vi "configuration UI.vi"() -> ()   [LabVIEW 2013, in "tag bus processing plugin editor node.lvclass"]
uses:
  tag bus processing plugin editor node.lvclass
  <vilib>/CEF_TreeControl/Node/NodeRef.ctl
  <vilib>/CEF_TreeControl/Node/NISE_CEF_Node.lvclass
  <vilib>/NI/AMC/Message Queue.ctl
  <vilib>/NI/AMC/Message.ctl
  <vilib>/NI/Tools/Keyed Array/KeyedArray.ctl
  <vilib>/CEF_TreeControl/Node/UserEventRef.ctl
  <vilib>/CEF_TreeControl/Controls/EventCluster.ctl
  module/configuration/tag bus processing plugin module configuration.lvclass
  module/configuration/processing channels.ctl
  <vilib>/NI/Tag Bus Module Framework/channel/TBM channel.lvclass
  <vilib>/NI/Tag Bus Module Framework/root configuration/TBM configuration.lvclass/TBM configuration.ctl
  Configuration Editor/Classes/Engine Parent/Engine Parent Editor Node.lvclass
  <vilib>/NI/Tag Bus Module Framework/root configuration/Read instance name.vi
  Configuration Editor/Classes/Module editor node/Read Module Configuration.vi
  <vilib>/NI/Tag Bus Module Framework/root configuration/create GUID.vi
  <vilib>/NI/Tag Bus Module Framework/module configuration/TBM module configuration.lvclass
  <vilib>/NI/Module Execution Interface/Engine Configuration/engine configuration.lvclass
  <vilib>/CEF_TreeControl/NISE_CEF_TreeControl.lvlib
  <vilib>/NI/Tools/Keyed Array/Tools_KeyedArray.lvlib
  <vilib>/NI/AMC/AMC.lvlib
panel:
  in  "Tab Control":enum32{"Control Configuration"}(tab)
  in  "delete":bool
  in  "add":bool
  in  "Result Tag":u16(ring)
  in  "Parameter Tag":u16(ring)
  in  "Functions":i32(listbox)
  in  "user event":T1
  in  "main queue":T2
  in  "node ref":T3
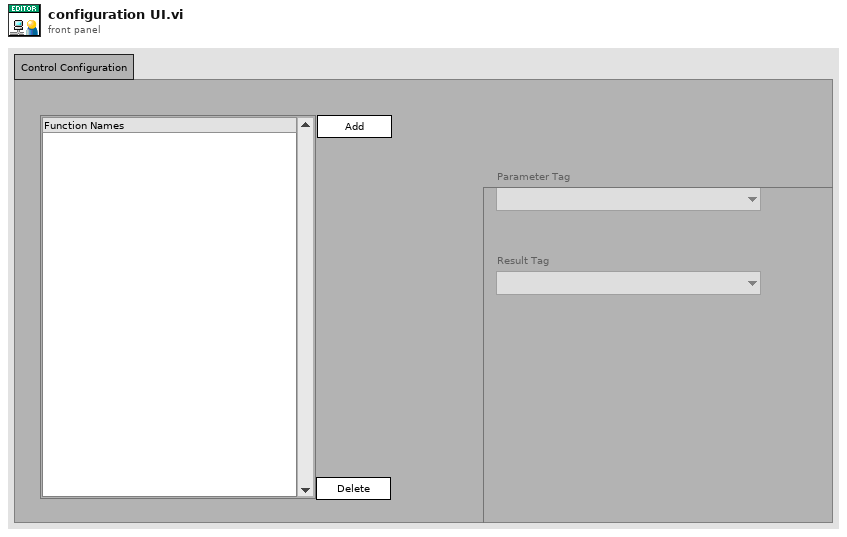
[diagram p1: front panel]
types:
  T1 = typedef "NISE_CEF_Node.lvclass/UserEventRef.ctl" = refnum<user-event>
  T2 = typedef "AMC.lvlib/Message Queue.ctl" = refnum<queue>
  T3 = typedef "NISE_CEF_Node.lvclass/NodeRef.ctl" = refnum<data-value>
  T4 = typedef "tag bus processing plugin module configuration.lvclass/processing channels.ctl" = cluster{"parameter":refnum<class "TBM channel.lvclass">, "result":refnum<class "TBM channel.lvclass">}
  T5 = typedef "NISE_CEF_TreeControl.lvlib/EventCluster.ctl" = cluster{"command":string, "data":string}
  T6 = enum8{"Enabled", "Disabled", "Disabled and Grayed Out"}
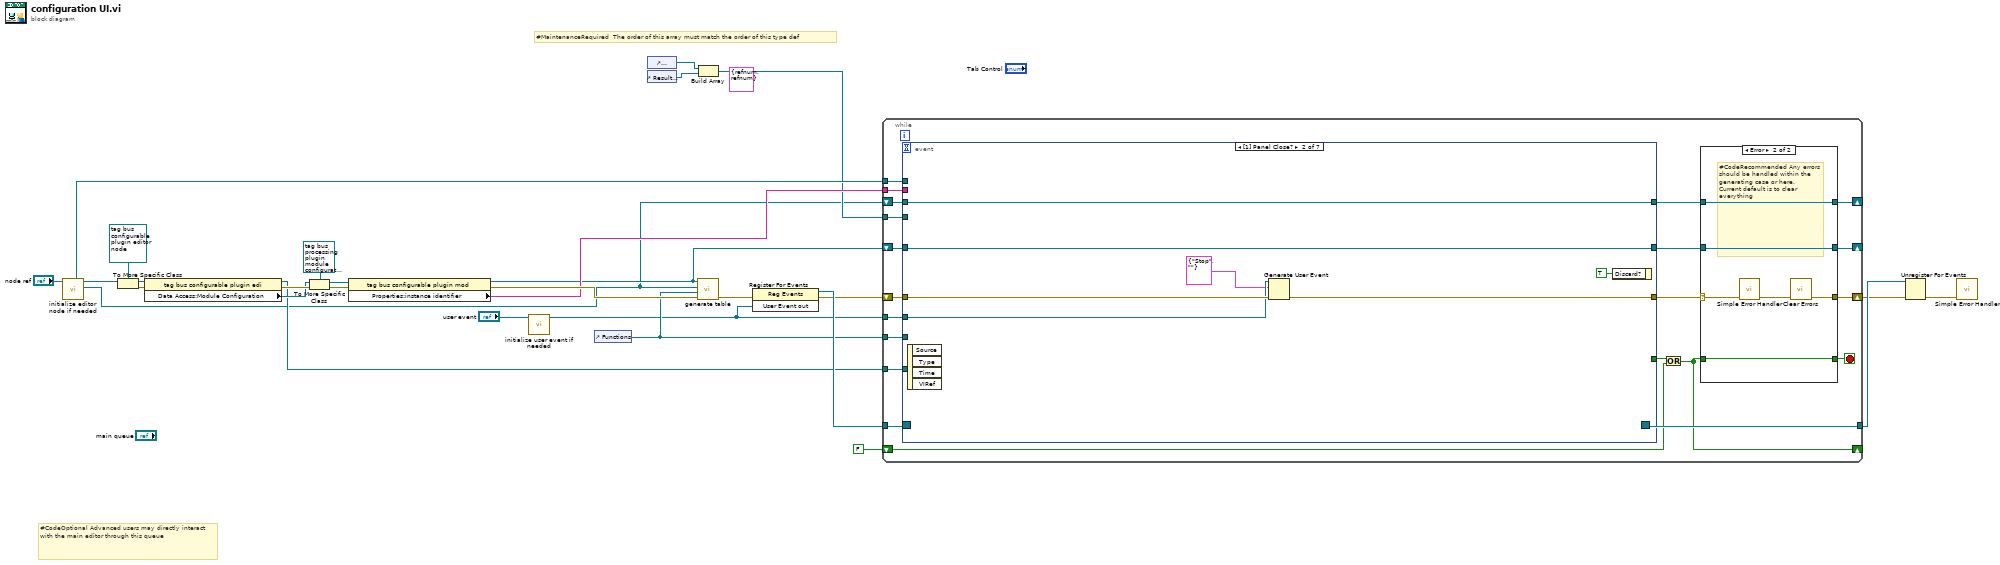
[diagram p0: block diagram]
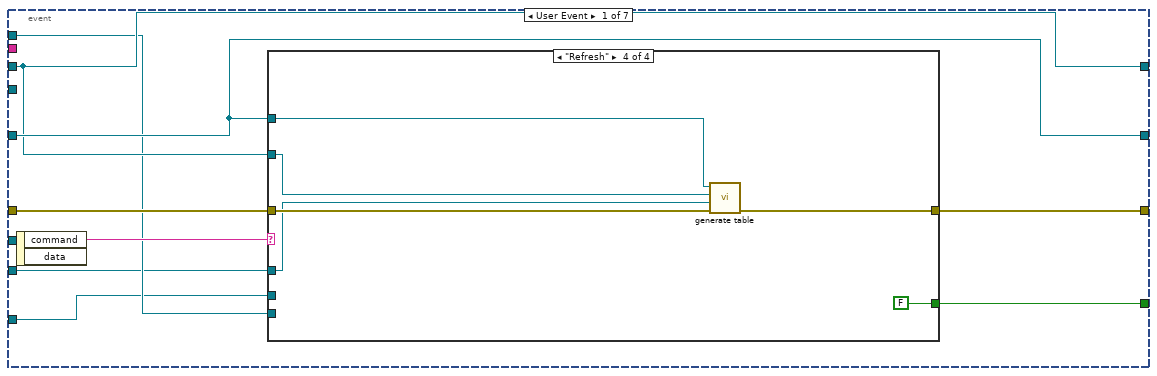
[diagram p3: hidden frame]
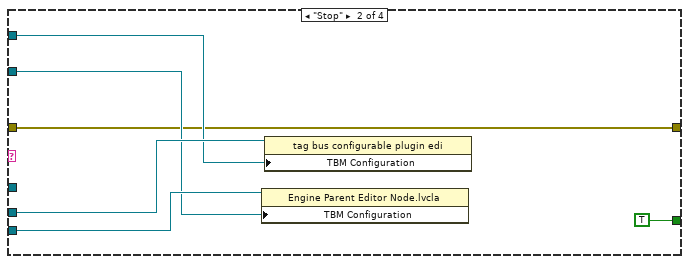
[diagram p5: hidden frame]
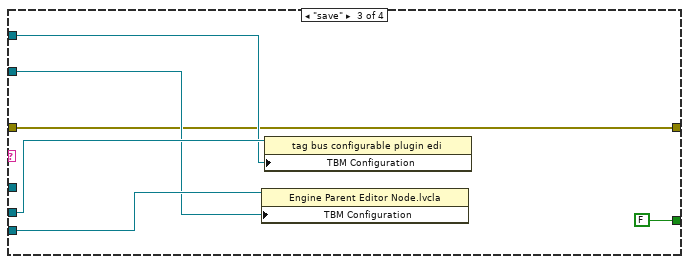
[diagram p6: hidden frame]
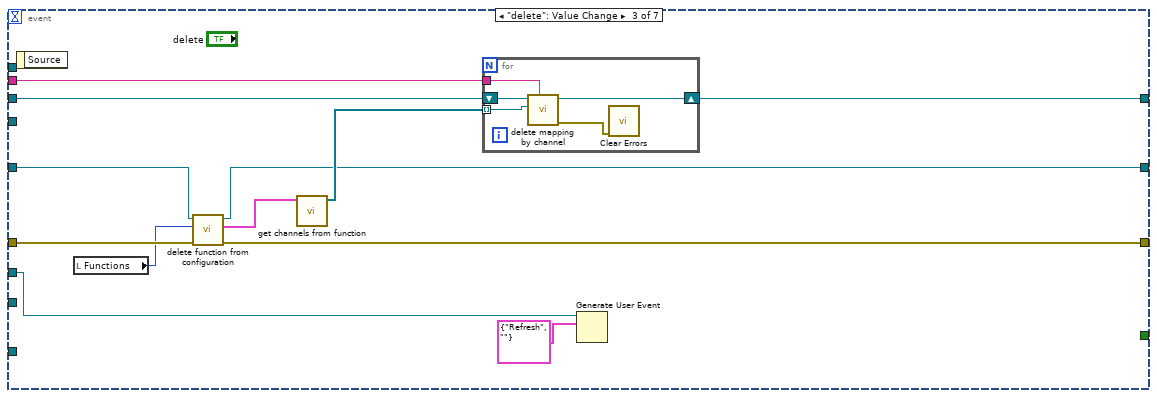
[diagram p7: hidden frame]
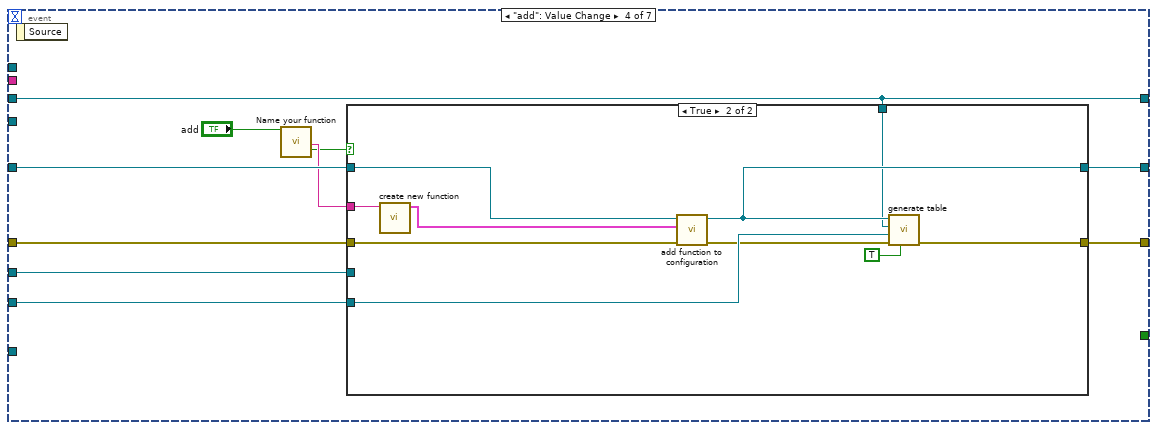
[diagram p8: hidden frame]
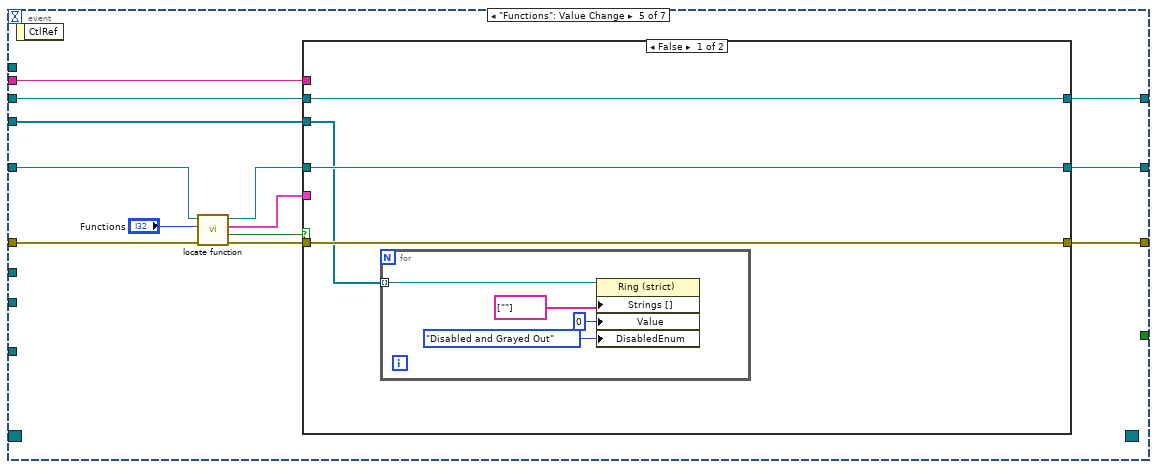
[diagram p10: hidden frame]
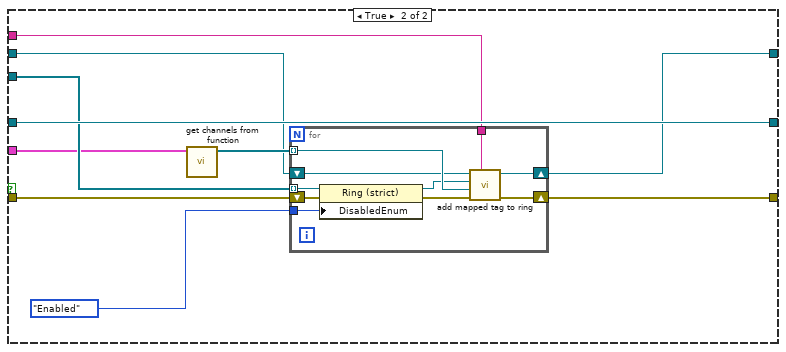
[diagram p11: hidden frame]
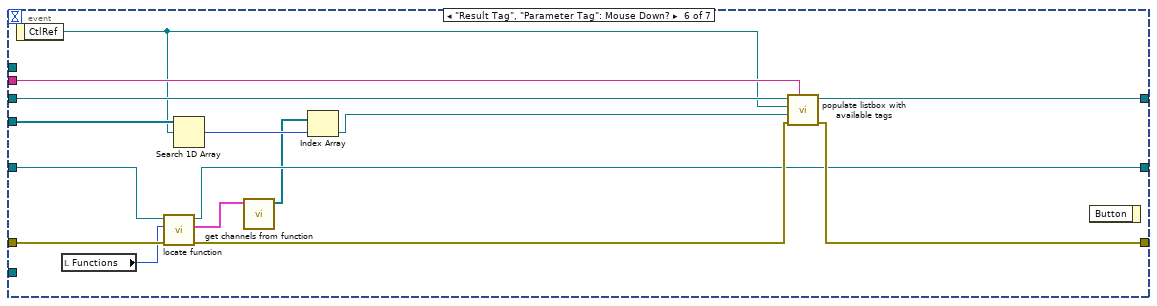
[diagram p12: hidden frame]
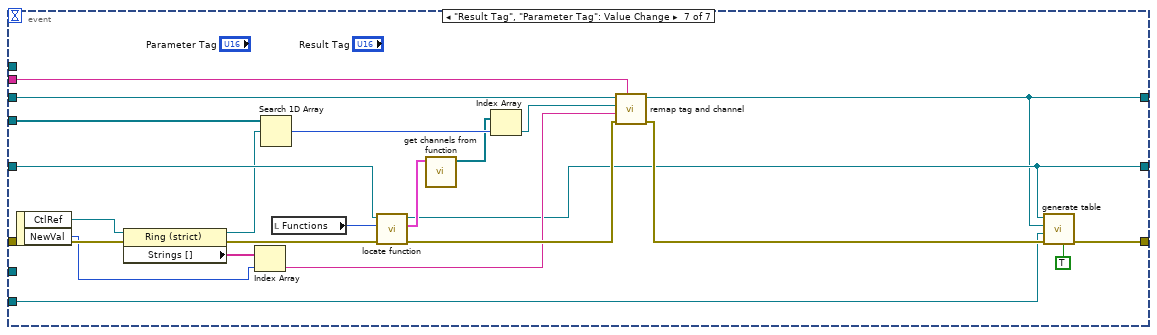
[diagram p13: hidden frame]
diagram:
  (unwired) T4 {"parameter"=refnum, "result"=refnum} ("processing function")
  # "#MaintenanceRequired  The order of this array must match the order of this type def"
  # "#CodeOptional Advanced users may directly interact with the main editor through this queue"
  n1 = call "initialize editor node if needed.vi"("editor node in"="node ref") -> ("Engine Configuration"=w1:refnum<class "engine configuration.lvclass">, "editor node out"=w21:T3, "engine"=w19:refnum<data-value>)  [unwired: 8 in]
  n2 = To More Specific Class(target class=refnum<data-value> refnum ("data value reference"), reference=w21) -> (specific class reference=w17:refnum<data-value>, error out=w16:errorcluster)  [unwired: 1 in]
  n3 = property class="tag bus configurable plugin edi"(reference=w17, error in=w16) -> (reference out=w7:refnum<data-value>, error out=w15:errorcluster, "Data Access:Module Configuration"=w14:refnum<class "TBM module configuration.lvclass">)
  n4 = To More Specific Class(target class=refnum<class "tag bus processing plugin module configuration.lvclass"> refnum ("tag bus configurable plugin module configuration"), reference=w14, error in=w15) -> (specific class reference=w11:refnum<class "tag bus processing plugin module configuration.lvclass">, error out=w12:errorcluster)
  n5 = property class="tag bus configurable plugin mod"(reference=w11, error in=w12) -> (reference out=w2:refnum<class "tag bus processing plugin module configuration.lvclass">, error out=w10:errorcluster, "Properties:instance identifier"=w9:string)
  n6 = call "initialize user event if needed.vi"("User Event in"="user event") -> ("User Event out"=w3:T1)  [unwired: 10 in]
  n7 = control-ref of="Functions"() -> (w8:refnum<vi>)
  n8 = control-ref of="Parameter Tag"() -> (w6:refnum<vi>)
  n9 = control-ref of="Result Tag"() -> (w5:refnum<vi>)
  n10 = call "generate table.vi"("error in"=w10, "listbox"=w8, "engine configuration in"=w1, "tag bus configurable plugin module configuration in"=w2) -> ("error out"=w24:errorcluster)  [unwired: 7 in]
  n11 = Build Array(w6, w5) -> (w4:refnum<vi>[])
  n12 = register-events(error in=w24, w3) -> (reference out=w29:refnum<event-registration>, error out=w23:errorcluster)  [unwired: 1 in]
  n13 = while {
    tunnel: w29 -> [w50]
    tunnel: [w49] -> w28
    shift-right: [w42] -> w27
    shift-left: w23 -> [w48]
    shift-right: [w44] -> _
    shift-left: FALSE -> [w43]
    shift-right: [w38] -> _
    shift-left: w1 -> [w41]
    shift-right: [w37] -> _
    shift-left: w2 -> [w40]
    tunnel: w9 -> [w35]
    tunnel: w8 -> [w34]
    tunnel: w4 -> [w33]
    tunnel: w7 -> [w32]
    tunnel: w19 -> [w31]
    tunnel: w3 -> [w30]
    stop <- w46 stop-if-true
    n14 = event shown="[1] Panel Close?" {
      selector: w50 -> [_ _ _ _ _ _ _]
      dyn-events: [_ _ _ _ _ _ _] -> w49
      timeout: _ -> [_ _ _ _ _ _ _]
      tunnel: [w66 _ _ _ _ _ _] -> w45
      tunnel: [w69 w92 w100 w122 w141 w187 w202] -> w47
      tunnel: w48 -> [w68 w95 w107 w119 w147 w186 w213]
      tunnel: [w64 w94 w98 w113 w138 w189 w191] -> w39
      tunnel: w41 -> [w64 w94 w103 w113 w137 w190 w210]
      tunnel: [w65 w93 w99 w121 w140 w183 w192] -> w36
      tunnel: w40 -> [w65 w93 w105 w118 w146 w184 w205]
      tunnel: w35 -> [_ _ w101 _ w136 w188 w209]
      tunnel: w34 -> [w61 _ _ w120 _ _ w201]
      tunnel: w33 -> [_ _ _ _ w135 w181 w198]
      tunnel: w32 -> [w62 _ _ _ _ _ _]
      tunnel: w31 -> [w63 _ _ _ _ _ _]
      tunnel: w30 -> [_ w91 w96 w114 _ _ _]
      event User Event {
        n15 = event-data() -> ("command"=w67:string)  [unwired: 1 in, 1 out]
        n16 = case shown="\"Refresh\"" w67 {
          tunnel: [_ TRUE FALSE FALSE] -> w66
          tunnel: w62 -> [_ w75 w81 _]
          tunnel: w63 -> [_ w74 w80 _]
          tunnel: w65 -> [_ w73 w79 w85]
          tunnel: w64 -> [_ w72 w78 w84]
          tunnel: w68 -> [w70 w71 w77 w87]
          tunnel: [w70 w71 w77 w86] -> w69
          tunnel: w61 -> [_ _ _ w83]
          frame Default {
          }
          frame "Stop" {
            n17 = property class="Engine Parent Editor Node.lvcla"(reference=w74, "TBM Configuration"=w72) -> ()  [unwired: 1 in, 2 out]
            n18 = property class="tag bus configurable plugin edi"(reference=w75, "TBM Configuration"=w73) -> ()  [unwired: 1 in, 2 out]
          }
          frame "save" {
            n19 = property class="Engine Parent Editor Node.lvcla"(reference=w80, "TBM Configuration"=w78) -> ()  [unwired: 1 in, 2 out]
            n20 = property class="tag bus configurable plugin edi"(reference=w81, "TBM Configuration"=w79) -> ()  [unwired: 1 in, 2 out]
          }
          frame "Refresh" {
            n21 = call "generate table.vi"("error in"=w87, "listbox"=w83, "engine configuration in"=w84, "tag bus configurable plugin module configuration in"=w85) -> ("error out"=w86:errorcluster)  [unwired: 7 in]
          }
        }
      }
      event Panel Close? {
        n22 = event-data() -> ()  [unwired: 1 in, 4 out]
        n23 = Generate User Event(user event=w91, event data cluster=T5 {"command"="Stop", "data"=""} ("event data"), error in=w95) -> (error out=w92:errorcluster)  [unwired: 1 in, 1 out]
        n24 = event-data("Discard?"=TRUE) -> ()  [unwired: 1 in, 1 out]
      }
      event "delete": Value Change {
        n25 = event-data() -> ()  [unwired: 1 in, 1 out]
        n26 = local read "Functions"() -> (w106:i32)
        n27 = call "delete function from configuration.vi"("error in"=w107, "index"=w106, "tag bus configurable plugin module configuration in"=w105) -> ("error out"=w100:errorcluster, "function deleted"=w104:T4, "tag bus configurable plugin module configuration out"=w99:refnum<class "tag bus processing plugin module configuration.lvclass">)  [unwired: 6 in]
        n28 = call "get channels from function.vi"("processing function"=w104) -> ("channels"=w102:refnum<class "TBM channel.lvclass">[])  [unwired: 10 in]
        n29 = for {
          shift-right: [w109] -> w98
          shift-left: w103 -> [w112]
          tunnel: w102 -> [w111] mode=indexing
          tunnel: w101 -> [w110]
          n30 = call <vilib>:"delete mapping by channel.vi"("owner ID"=w110, "channel"=w111, "engine configuration in"=w112) -> ("error out"=w108:errorcluster, "engine configuration out"=w109:refnum<class "engine configuration.lvclass">)  [unwired: 7 in]
          n31 = call <vilib>:"Clear Errors.vi"("error in (no error)"=w108) -> ()  [unwired: 6 in, 1 out]
        }
        n32 = Generate User Event(user event=w96, event data cluster=T5 {"command"="Refresh", "data"=""} ("event data")) -> ()  [unwired: 2 in, 2 out]
      }
      event "add": Value Change {
        n33 = event-data() -> ()  [unwired: 1 in, 1 out]
        n34 = call "Name your function"("Enable"="add") -> ("function name"=w117:string, "OK"=w116:bool)  [unwired: 16 in, 1 out]
        n35 = case shown="True" w116 {
          tunnel: [w123 w134] -> w122
          tunnel: [w124 w126] -> w121
          tunnel: w120 -> [_ w133]
          tunnel: w119 -> [w123 w132]
          tunnel: w118 -> [w124 w131]
          tunnel: w117 -> [_ w128]
          tunnel: w114 -> [_ _]
          tunnel: w113 -> [_ w125]
          frame False {
          }
          frame True {
            n36 = call "create new function.vi"("function name"=w128) -> ("processing function"=w127:T4)  [unwired: 10 in]
            n37 = call "add function to configuration.vi"("error in"=w132, "processing function"=w127, "tag bus configurable plugin module configuration in"=w131) -> ("error out"=w130:errorcluster, "tag bus configurable plugin module configuration out"=w126:refnum<class "tag bus processing plugin module configuration.lvclass">)  [unwired: 7 in]
            n38 = call "generate table.vi"("select last?"=TRUE, "error in"=w130, "listbox"=w133, "engine configuration in"=w125, "tag bus configurable plugin module configuration in"=w126) -> ("error out"=w134:errorcluster)  [unwired: 6 in]
          }
        }
      }
      event "Functions": Value Change {
        n39 = event-data() -> ()  [unwired: 1 in, 1 out]
        n40 = call "locate function.vi"("error in"=w147, "index"="Functions", "tag bus processing plugin module configuration in"=w146) -> ("error out"=w142:errorcluster, "found"=w144:bool, "processing function"=w145:T4, "tag bus processing plugin module configuration out"=w139:refnum<class "tag bus processing plugin module configuration.lvclass">)  [unwired: 5 in]
        n41 = case shown="False" w144 {
          tunnel: w145 -> [_ w162]
          tunnel: w142 -> [w149 w161]
          tunnel: [w149 w157] -> w141
          tunnel: [w150 w165] -> w140
          tunnel: w139 -> [w150 w165]
          tunnel: [w151 w158] -> w138
          tunnel: w137 -> [w151 w156]
          tunnel: w136 -> [_ w159]
          tunnel: w135 -> [w148 w163]
          frame False {
            n42 = for {
              tunnel: w148 -> [w152] mode=indexing
              n43 = property on="Property Node" class="Ring (strict)"(reference=w152, "Strings []"=string[] [""], "Value"=u16 0, "DisabledEnum"=T6."Disabled and Grayed Out" ("Disabled")) -> ()  [unwired: 1 in, 2 out]
            }
          }
          frame True {
            n44 = call "get channels from function.vi"("processing function"=w162) -> ("channels"=w160:refnum<class "TBM channel.lvclass">[])  [unwired: 10 in]
            n45 = for {
              tunnel: T6."Enabled" ("Disabled") -> [w175]
              tunnel: w163 -> [w174] mode=indexing
              shift-right: [w171] -> w157
              shift-left: w161 -> [w173]
              tunnel: w160 -> [w170] mode=indexing
              tunnel: w159 -> [w168]
              shift-right: [w166] -> w158
              shift-left: w156 -> [w167]
              n46 = property on="Property Node" class="Ring (strict)"(reference=w174, error in=w173, "DisabledEnum"=w175) -> (reference out=w169:refnum<vi>, error out=w172:errorcluster)
              n47 = call "add mapped tag to ring.vi"("instance id"=w168, "error in"=w172, "channel"=w170, "ring"=w169, "engine configuration in"=w167) -> ("error out"=w171:errorcluster, "engine configuration out"=w166:refnum<class "engine configuration.lvclass">)  [unwired: 4 in, 1 out]
            }
          }
        }
      }
      event "Result Tag", "Parameter Tag": Mouse Down? {
        n48 = event-data() -> ("CtlRef"=w180:refnum<vi>)  [unwired: 1 in]
        n49 = local read "Functions"() -> (w182:i32)
        n50 = call "locate function.vi"("error in"=w186, "index"=w182, "tag bus processing plugin module configuration in"=w184) -> ("error out"=w185:errorcluster, "processing function"=w179:T4, "tag bus processing plugin module configuration out"=w183:refnum<class "tag bus processing plugin module configuration.lvclass">)  [unwired: 5 in, 1 out]
        n51 = Search 1D Array(1D array=w181, element=w180) -> (index of element=w178:i32)  [unwired: 1 in]
        n52 = call "get channels from function.vi"("processing function"=w179) -> ("channels"=w177:refnum<class "TBM channel.lvclass">[])  [unwired: 10 in]
        n53 = Index Array(array=w177, index=w178) -> (element=w176:refnum<class "TBM channel.lvclass">)
        n54 = call "populate listbox with available tags.vi"("instance id"=w188, "error in"=w185, "channel"=w176, "CtlRef"=w180, "engine configuration in"=w190) -> ("error out"=w187:errorcluster, "engine configuration out"=w189:refnum<class "engine configuration.lvclass">)  [unwired: 5 in]
        n55 = event-data() -> ()  [unwired: 2 in, 1 out]
      }
      event "Result Tag", "Parameter Tag": Value Change {
        n56 = event-data() -> ("CtlRef"=w212:refnum<vi>, "NewVal"=w199:u16)  [unwired: 1 in]
        n57 = property class="Ring (strict)"(reference=w212, error in=w213) -> (reference out=w197:refnum<vi>, error out=w206:errorcluster, "Strings []"=w211:string[])
        n58 = Index Array(array=w211, index=w199) -> (element=w204:string)
        n59 = Search 1D Array(1D array=w198, element=w197) -> (index of element=w195:i32)  [unwired: 1 in]
        n60 = local read "Functions"() -> (w208:i32)
        n61 = call "locate function.vi"("error in"=w206, "index"=w208, "tag bus processing plugin module configuration in"=w205) -> ("error out"=w207:errorcluster, "processing function"=w196:T4, "tag bus processing plugin module configuration out"=w192:refnum<class "tag bus processing plugin module configuration.lvclass">)  [unwired: 5 in, 1 out]
        n62 = call "get channels from function.vi"("processing function"=w196) -> ("channels"=w194:refnum<class "TBM channel.lvclass">[])  [unwired: 10 in]
        n63 = Index Array(array=w194, index=w195) -> (element=w193:refnum<class "TBM channel.lvclass">)
        n64 = call "remap tag and channel.vi"("instance id"=w209, "error in"=w207, "tag name"=w204, "channel"=w193, "engine configuration in"=w210) -> ("error out"=w203:errorcluster, "engine configuration out"=w191:refnum<class "engine configuration.lvclass">)  [unwired: 5 in]
        n65 = call "generate table.vi"("only redraw current"=TRUE, "error in"=w203, "listbox"=w201, "engine configuration in"=w191, "tag bus configurable plugin module configuration in"=w192) -> ("error out"=w202:errorcluster)  [unwired: 6 in]
      }
    }
    n66 = Or(x=w45, y=w43) -> (x .or. y?=w44:bool)
    n67 = case shown="Error" w47 {
      selector: w47 -> [w53 w59]
      tunnel: [w54 w60] -> w46
      tunnel: w44 -> [w54 w60]
      tunnel: [w53 w57] -> w42
      tunnel: w39 -> [w52 w55]
      tunnel: [w52 w55] -> w38
      tunnel: [w51 w56] -> w37
      tunnel: w36 -> [w51 w56]
      frame No Error {
      }
      frame Error {
        # "#CodeRecommended Any errors should be handled within the generating case or here. Current default is to clear everything"
        n68 = call <vilib>:"Simple Error Handler.vi"("error in (no error)"=w59) -> ("error out"=w58:errorcluster)  [unwired: 4 in, 4 out]
        n69 = call <vilib>:"Clear Errors.vi"("error in (no error)"=w58) -> ("error out"=w57:errorcluster)  [unwired: 6 in]
      }
    }
  }
  n70 = Unregister For Events(event registration refnum=w28, error in=w27) -> (error out=w18:errorcluster)
  n71 = call <vilib>:"Simple Error Handler.vi"("error in (no error)"=w18) -> ()  [unwired: 4 in, 5 out]
